vi "GetPointType2D_3D-DBL.vi"(11 "Point":T1) -> (3 "Point":T2)   [LabVIEW 2020, in "OpenLvVision_OpenCv.lvlib"]
uses:
  TypeDef/Point/2D_PointDBL.ctl
  OpenLvVision_OpenCv.lvlib
  TypeDef/Point/3D_PointDBL.ctl
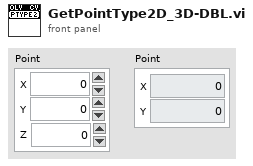
[diagram p1: front panel]
types:
  T1 = typedef "OpenLvVision_OpenCv.lvlib/3D_PointDBL.ctl" = cluster{"X":dbl, "Y":dbl, "Z":dbl}
  T2 = typedef "OpenLvVision_OpenCv.lvlib/2D_PointDBL.ctl" = cluster{"X":dbl, "Y":dbl}
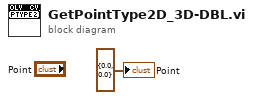
[diagram p0: block diagram]
diagram:
  "Point" <- T2 {"X"=0.0, "Y"=0.0} ("Point")
